vi "GetNumCamFrames.vi"(9 "Digital Waveform Graph":digitalwaveform[](array[waveform]), 10 "DO ports":cluster{"Camera trigger":tag}, 11 "Digital Used Lines":tag[](array[tag])) -> (3 "Numeric":i32)   [LabVIEW 2015]
uses:
  <vilib>/Waveform/DWDTOps.llb/DWDT Digital to Boolean Array.vi
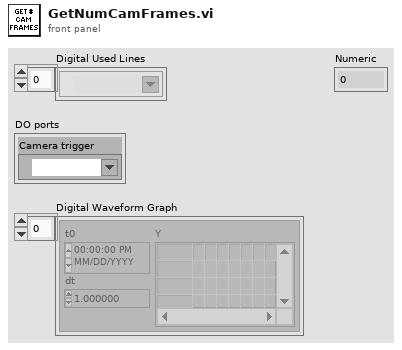
[diagram p1: front panel]
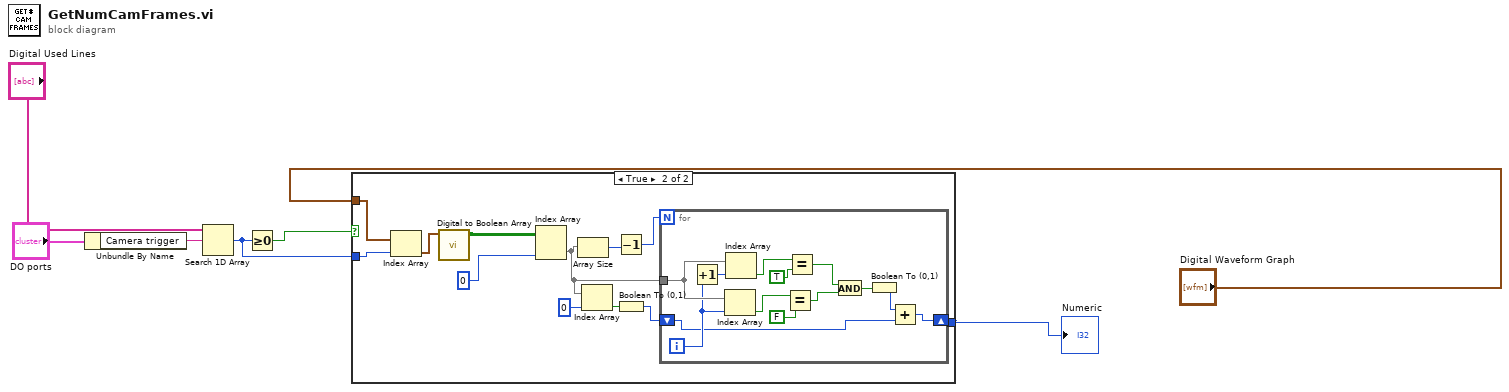
[diagram p0: block diagram]
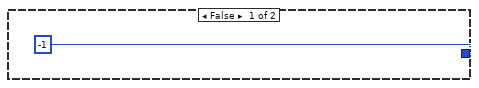
[diagram p2: hidden frame]
diagram:
  n1 = Unbundle By Name("DO ports") -> ("Camera trigger"=w5:tag)
  n2 = Search 1D Array(1D array="Digital Used Lines", element=w5) -> (index of element=w3:i32)  [unwired: 1 in]
  n3 = Greater Or Equal To 0?(x=w3) -> (x >= 0?=w1:bool)
  n4 = case shown="True" w1 {
    tunnel: "Digital Waveform Graph" -> [_ w19]
    tunnel: w3 -> [_ w20]
    tunnel: [-1 w14] -> w6
    frame False {
    }
    frame True {
      n5 = Index Array(array=w19, index=w20) -> (element=w16:digitalwaveform)
      n6 = call-poly <vilib>:"Digital to Boolean Array.vi"("digital waveform"=w16) -> ("boolean array"=w15:bool[][])  [unwired: 9 in, 1 out]
      n7 = Index Array(array=w15, index (col)=0) -> (element=w13:bool[])  [unwired: 1 in]
      n8 = Array Size(array=w13) -> (size(s)=w17:i32)
      n9 = Index Array(array=w13, index=0) -> (element=w11:bool)
      n10 = Decrement(x=w17) -> (x-1=w18:i32)
      n11 = Boolean To (0,1)(Boolean=w11) -> (0, 1=w10:i16)
      n12 = for {
        N: w18 -> [_]
        tunnel: w13 -> [w33]
        shift-right: [w21] -> w14
        shift-left: w10 -> [w22]
        i -> [w31]
        n13 = Increment(x=w31) -> (x+1=w32:i32)
        n14 = Index Array(array=w33, index=w31) -> (element=w29:bool)
        n15 = Index Array(array=w33, index=w32) -> (element=w27:bool)
        n16 = Equal?(x=w29, y=FALSE) -> (x = y?=w25:bool)
        n17 = Equal?(x=w27, y=TRUE) -> (x = y?=w26:bool)
        n18 = And(x=w26, y=w25) -> (x .and. y?=w24:bool)
        n19 = Boolean To (0,1)(Boolean=w24) -> (0, 1=w23:i16)
        n20 = Add(x=w23, y=w22) -> (x+y=w21:i16)
      }
    }
  }
  "Numeric" <- w6
